vi "_New.vi"(8 "error in (no error)":errorcluster) -> (0 "error out":errorcluster, 3 "JMETestSolutions.Instrument.DMM out":refnum<class "JMETestSolutions.Instrument.DMM.lvclass">)   [LabVIEW 2020]
uses:
  JMETestSolutions.Instrument.DMM.lvclass
panel:
  in  "JMETestSolutions.Instrument.DMM in":refnum<class "JMETestSolutions.Instrument.DMM.lvclass">
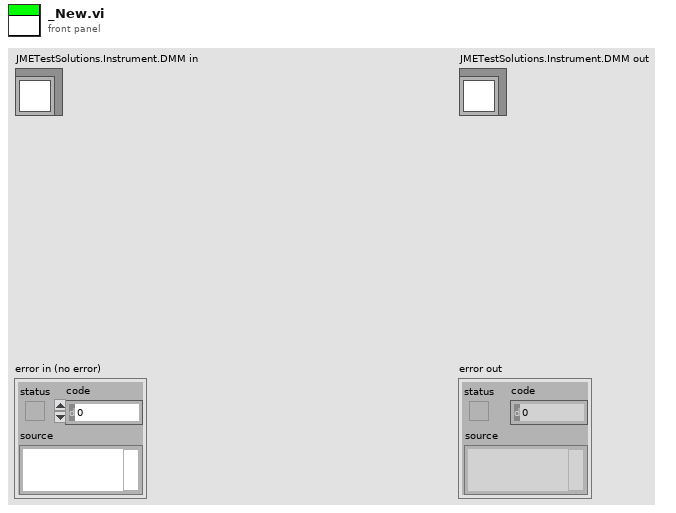
[diagram p1: front panel]
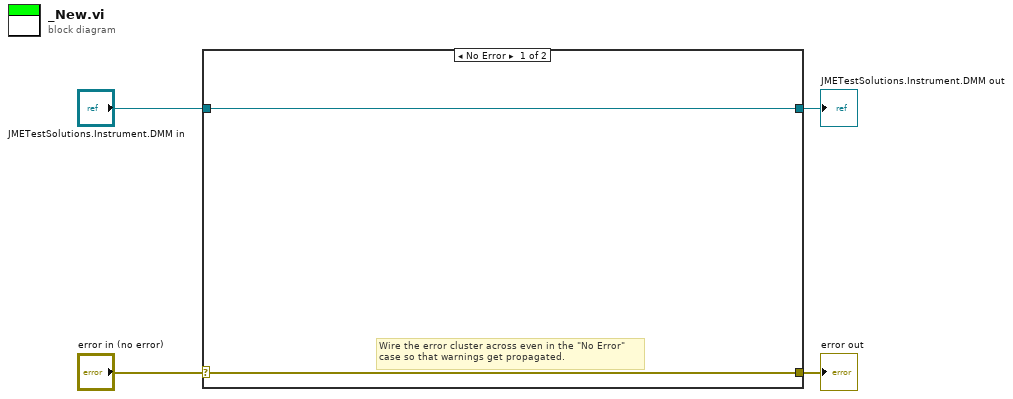
[diagram p0: block diagram]
diagram:
  n1 = case shown="No Error" "error in (no error)" {
    selector: "error in (no error)" -> [w5 w8]
    tunnel: [w5 w8] -> w3
    tunnel: [w6 w7] -> w1
    tunnel: "JMETestSolutions.Instrument.DMM in" -> [w6 w7]
    frame No Error {
      # "Wire the error cluster across even in the \"No Error\"\ncase so that warnings get propagated."
    }
    frame Error {
    }
  }
  "error out" <- w3
  "JMETestSolutions.Instrument.DMM out" <- w1
